vi "火车故障检测系统.vi"() -> ()   [LabVIEW 2015]
doc: "仿真实际的逐点应用。根据仿真实时数据采集和分析，检测火车轮的故障。每列火车包含6个车轮，它们分别由仿真数据图表中的突波表示。突波的高度可确定车轮是否正常。每辆火车传递至底部的条形图，可显示车轮是否正常。"
uses:
  <vilib>/Analysis/3filter.llb/Filter Passband Type.ctl
  <vilib>/ptbypt/NI_PtbyPt.lvlib
  <vilib>/Analysis/NI_AALBase.lvlib
panel:
  out "检测的火车":bool
  out "阈值数据":dbl(graph)
  out "仿真数据（8列火车）":cluster{"Filtered x":dbl, dbl, "threshold":dbl}(graph)
  out "坏/好的车轮":dbl[](graph)
  out "火车数量":u32
  out "检测到的车轮":bool
  out "车轮数量":u32
  in  "滤波器阶数":i32=4
  in  "低频":dbl=0.01 format="%#.6g"
  in  "窗长度":i32=100
  in  "阈值":dbl(slide)=15.0 scale=-10.0..40.0
  in  "高频":dbl=0.25 format="%#.6g"
  in  "仿真速度":u32(slide)=5 scale=1.0..10.0
  in  "停止":bool
  # "滤波器参数"
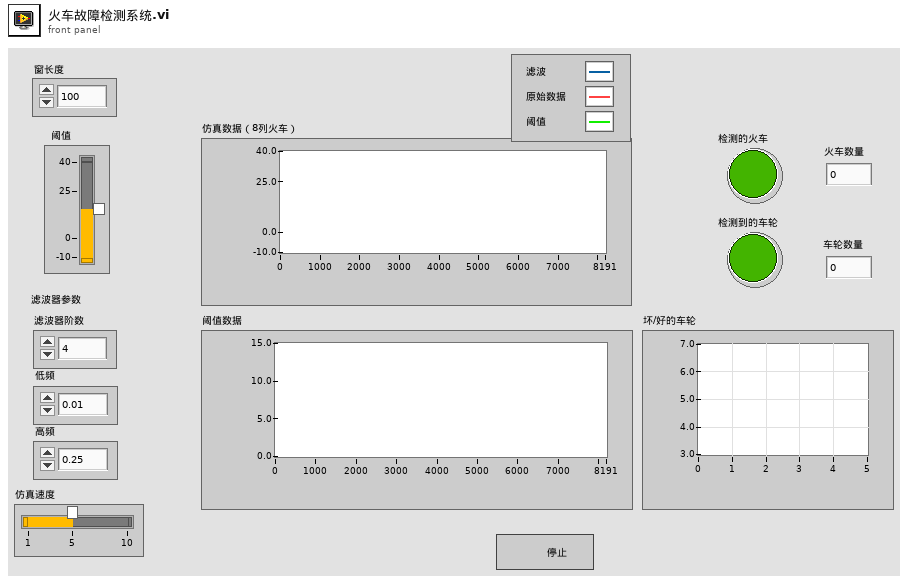
[diagram p1: front panel]
types:
  T1 = cluster{dbl, "Filtered x":dbl, "Filtered x 2":dbl}[]
  T2 = typedef "NI_AALBase.lvlib/Filter Passband Type.ctl" = enum32{"Lowpass", "Highpass", "Bandpass", "Bandstop"}
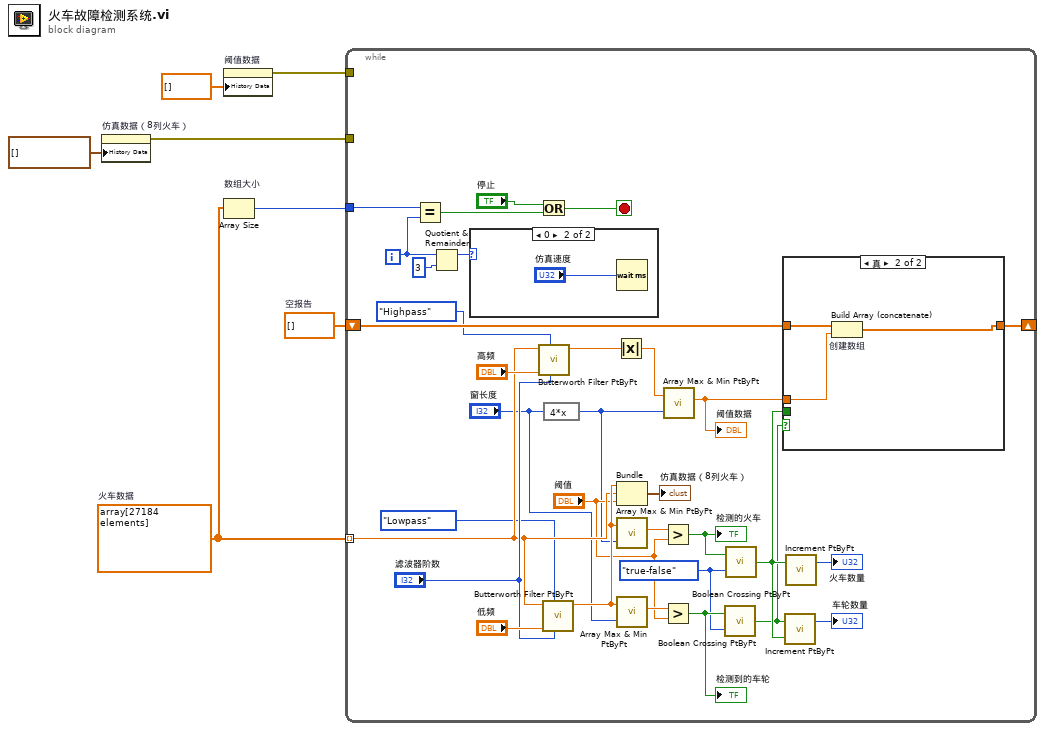
[diagram p0: block diagram]
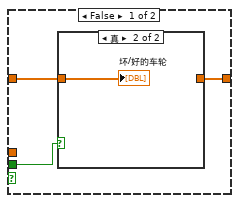
[diagram p3: hidden frame]
diagram:
  w5 = dbl[] array[27184 elements]  # 火车数据
  w7 = dbl[] []  # 空报告
  n1 = property on="仿真数据（8列火车）" class="WFChart (严格)"("History Data"=T1 []) -> (error out=w1:errorcluster)  [unwired: 2 in, 1 out]
  n2 = property on="阈值数据" class="WFChart (严格)"("History Data"=dbl[] []) -> (error out=w4:errorcluster)  [unwired: 2 in, 1 out]
  n3 = Array Size "数组大小"(array=w5) -> (size(s)=w6:i32)
  n4 = while {
    shift-left: w7 -> [w34]
    shift-right: [w35] -> _
    tunnel: w5 -> [w20] mode=indexing
    tunnel: w4 -> [_]
    tunnel: w6 -> [w29]
    tunnel: w1 -> [_]
    i -> [w28]
    stop <- w30 stop-if-true
    w8 = enum16{"either", "false-true", "true-false"}."true-false" ("direction")
    # "检测火车车轮故障"
    n5 = Equal?(x=w29, y=w28) -> (x = y?=w24:bool)
    n6 = Quotient & Remainder(x=w28, y=3) -> (x-y*floor(x/y)=w26:i32)  [unwired: 1 out]
    n7 = case shown="0" w26 {
      frame Default {
      }
      frame 0 {
        n8 = Wait (ms)(milliseconds to wait="仿真速度") -> ()  [unwired: 1 out]
      }
    }
    n9 = Or(x="停止", y=w24) -> (x .or. y?=w30:bool)
    n10 = call <vilib>:"Butterworth Filter PtByPt.vi"("order"="滤波器阶数", "filter type"=Filter_Passband_Type."Highpass", "low cutoff freq: fl"="高频", "x"=w20) -> ("Filtered x"=w12:dbl)  [unwired: 5 in, 1 out]
    n11 = call <vilib>:"Butterworth Filter PtByPt.vi"("order"="滤波器阶数", "filter type"=Filter_Passband_Type."Lowpass", "low cutoff freq: fl"="低频", "x"=w20) -> ("Filtered x"=w21:dbl)  [unwired: 5 in, 1 out]
    n12 = expression code="4*x" ("表达式节点")("窗长度") -> (w13:i32)
    n13 = Absolute Value(x=w12) -> (abs(x)=w22:dbl)
    n14 = Bundle ("捆绑")("Filtered x"=w21, w20, "阈值"="阈值") -> (→"仿真数据（8列火车）":cluster{"Filtered x":dbl, dbl, "阈值":dbl})  [unwired: 1 in]
    n15 = call <vilib>:"Array Max & Min PtByPt.vi"("input data point"=w21, "sample length"=w13) -> ("max value"=w33:dbl)  [unwired: 1 in, 4 out]
    n16 = call <vilib>:"Array Max & Min PtByPt.vi"("input data point"=w21, "sample length"="窗长度") -> ("max value"=w36:dbl)  [unwired: 1 in, 4 out]
    n17 = Greater?(x=w33, y="阈值") -> (0:w16:bool)
    "检测的火车" <- w16
    n18 = Greater?(x=w36, y="阈值") -> (0:w15:bool)
    "检测到的车轮" <- w15
    n19 = call <vilib>:"Array Max & Min PtByPt.vi"("input data point"=w22, "sample length"=w13) -> ("max value"=w11:dbl)  [unwired: 1 in, 4 out]
    "阈值数据" <- w11
    n20 = call <vilib>:"Boolean Crossing PtByPt.vi"("direction"=w8, "input"=w15) -> ("crossing"=w17:bool)  [unwired: 1 in]
    n21 = call <vilib>:"Boolean Crossing PtByPt.vi"("direction"=w8, "input"=w16) -> ("crossing"=w18:bool)  [unwired: 1 in]
    n22 = case shown="真" w17 {
      tunnel: w11 -> [_ w46]
      tunnel: w18 -> [w43 _]
      tunnel: [w42 w47] -> w35
      tunnel: w34 -> [w41 w48]
      frame False {
        n23 = case shown="真" w43 {
          tunnel: [w44 _] -> w42
          tunnel: w41 -> [w44 w45]
          frame False {
          }
          frame True {
            "坏/好的车轮" <- w45
          }
        }
      }
      frame True {
        n24 = Build Array (concatenate) "创建数组"(w48, w46) -> (w47:dbl[])
      }
    }
    n25 = call <vilib>:"Increment PtByPt.vi"("initialize"=w18, "activate"=w17) -> ("counter"=→"车轮数量":u32)  [unwired: 1 out]
    n26 = call <vilib>:"Increment PtByPt.vi"("activate"=w18) -> ("counter"=→"火车数量":u32)  [unwired: 1 in, 1 out]
  }
